vi "SMR_LabVIEW_V7.1.vi"() -> ()   [LabVIEW 2025]
uses:
  <vilib>/DAQmx/write.llb/DAQmx Write (Analog DBL 1Chan 1Samp).vi
  <vilib>/DAQmx/read.llb/DAQmx Read (Analog 1D DBL NChan 1Samp).vi
  <vilib>/DAQmx/create/channels.llb/DAQmx Create Channel (AI-Temperature-Thermocouple).vi
  <vilib>/DAQmx/create/channels.llb/DAQmx Create Channel (AI-Voltage-Basic).vi
  <vilib>/DAQmx/create/channels.llb/DAQmx Create Channel (AO-Voltage-Basic).vi
  <vilib>/DAQmx/miscellaneous.llb/DAQmx Fill In Error Info.vi
  <vilib>/addons/control/pid/pid.llb/PID (DBL).vi
  <vilib>/addons/control/pid/NI_PID_pid.lvlib
panel:
  out "Final P-Valve Voltage (V)":dbl
  out "PID Trim Voltage (V)":dbl
  in  "PID Temp Setpoint (deg C)":dbl
  in  "Auto PID Enable":bool
  in  "Manual P-Valve Voltage (V)":dbl min=0.0 max=10.0
  out "Rate Window Ready":bool
  out "Steady State":bool
  in  "Steady State Threshold (deg C/min)":dbl=0.5
  out "Temp Change Rate (deg C/min)":dbl
  in  "Voltage Limit (V)":dbl=10.0
  in  "Temperature Limit (C)":dbl=50.0
  in  "Pressure Limit (psi)":dbl=15.0
  out "Max Voltage":bool
  out "Max Temperature":bool
  out "Max Pressure":bool
  out "Current Run Folder":path
  in  "Log Root Folder":path=path "C:/Users/LocalUser/Documents/GitHub/thermal-loop/resources/v0.1.1/data/001"
  out "Heat Exchanger Pressure History":dbl(graph)
  out "Main Loop Pressure History":T1(graph)
  out "Heat Exchanger Temperature History":cluster{"Waveform":dbl, "Waveform":dbl}(graph)
  out "Main Loop Temeperature History":T2(graph)
  out "Overall Avg Pressure (psi)":dbl
  out "Heat Exchanger Pressure P6 (psi)":dbl
  out "Main Loop Avg Pressure (psi)":dbl
  out "Heat Exchanger Avg Temp (deg C)":dbl
  out "Main Loop Avg Temp (deg C)":dbl
  out "Raw NI9201 \nVoltage Display":T3
  out "Temperature Display":T4
  out "Pressure Display":T5
  in  "Flow Offset Correction (GPM)":dbl=-0.3
  out "Flow History":dbl(graph)
  out "Overall Pressure History":T6(graph)
  out "Overall Temperature History":T7(graph)
  out "Max Loop Pressure (psi)":dbl
  out "Overall Avg Temp (deg C)":dbl
  out "Max Loop Temp (deg C)":dbl
  out "Heat Exchanger Flow (GPM)":dbl
  in  "Loop Period (ms)":dbl=1000.0
  in  "Stop":bool
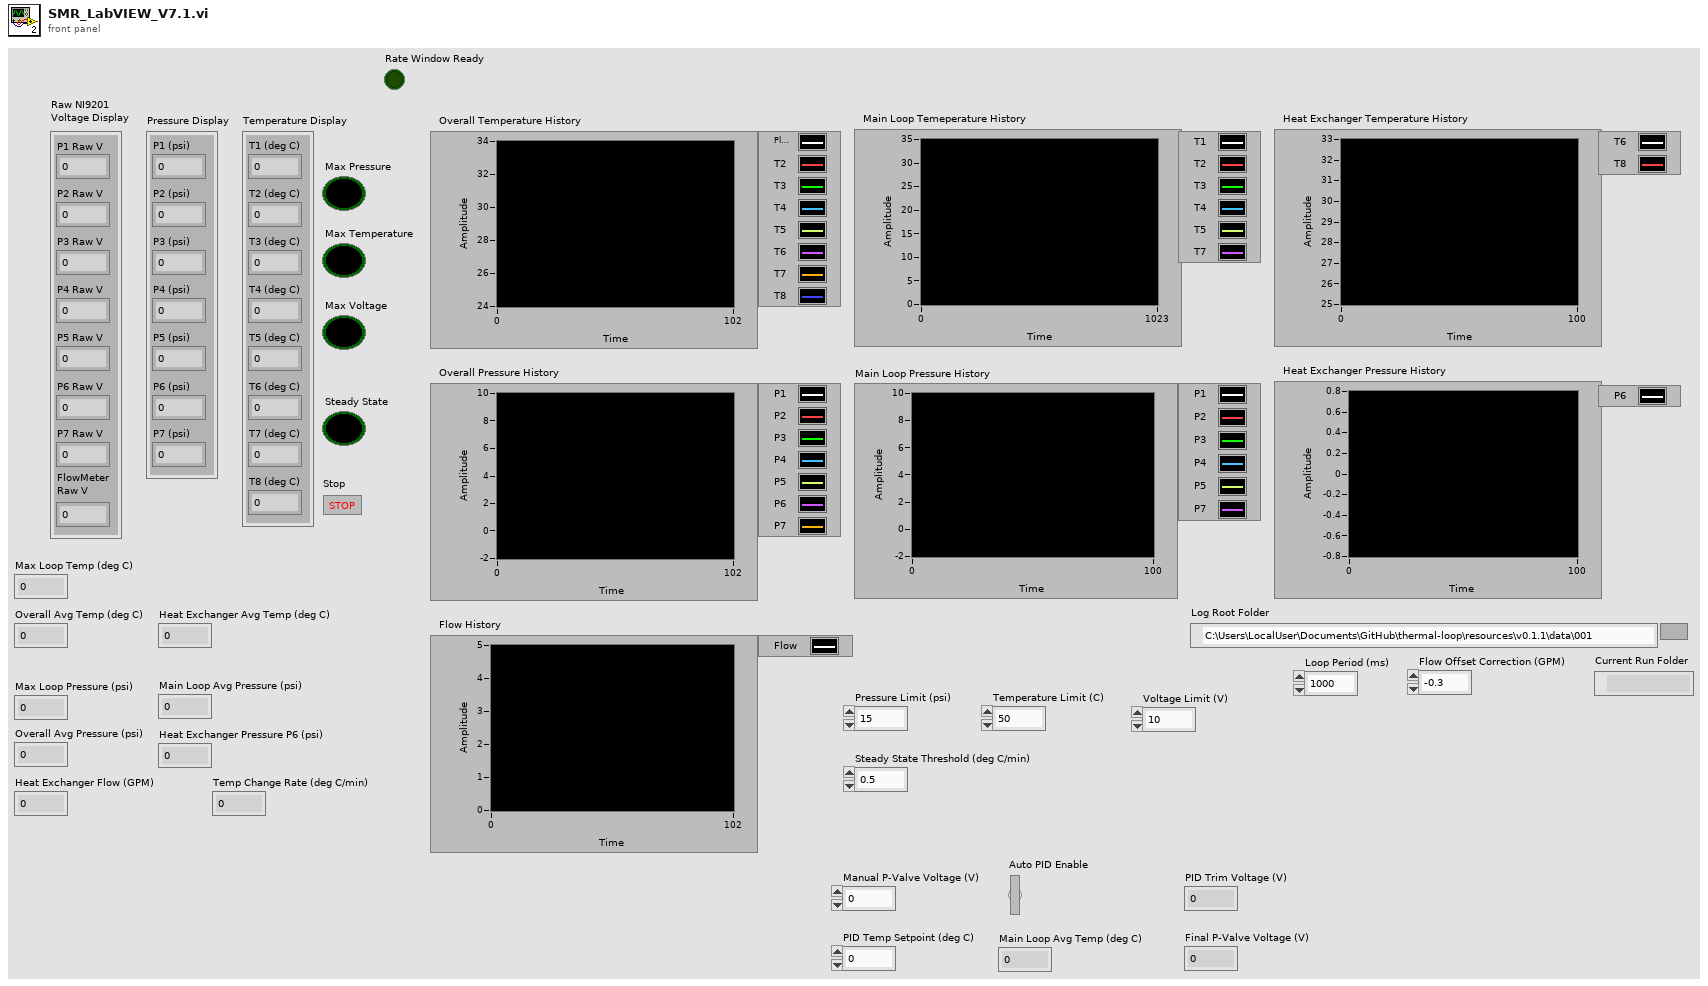
[diagram p1: front panel]
types:
  T1 = cluster{"P1":dbl, "P2":dbl, "P3":dbl, "P4":dbl, "P5":dbl, "P7":dbl}
  T2 = cluster{"Waveform":dbl, "Waveform":dbl, "Waveform":dbl, "Waveform":dbl, "Waveform":dbl, "Waveform":dbl}
  T3 = cluster{"P1 Raw V":dbl, "P2 Raw V":dbl, "P3 Raw V":dbl, "P4 Raw V":dbl, "P5 Raw V":dbl, "P6 Raw V":dbl, "P7 Raw V":dbl, "FlowMeter\nRaw V":dbl}
  T4 = cluster{"T1 (deg C)":dbl, "T2 (deg C)":dbl, "T3 (deg C)":dbl, "T4 (deg C)":dbl, "T5 (deg C)":dbl, "T6 (deg C)":dbl, "T7 (deg C)":dbl, "T8 (deg C)":dbl}
  T5 = cluster{"P1 (psi)":dbl, "P2 (psi)":dbl, "P3 (psi)":dbl, "P4 (psi)":dbl, "P5 (psi)":dbl, "P6 (psi)":dbl, "P7 (psi)":dbl}
  T6 = cluster{"P1":dbl, "P2":dbl, "P3":dbl, "P4":dbl, "P5":dbl, "P6":dbl, "P7":dbl}
  T7 = cluster{"Waveform":dbl, "Waveform":dbl, "Waveform":dbl, "Waveform":dbl, "Waveform":dbl, "Waveform":dbl, "Waveform":dbl, "Waveform":dbl}
  T8 = enum16{"open", "replace", "create", "open or create", "replace or create", "replace or create with confirmation"}
  T9 = cluster{"proportional gain (Kc)":dbl, "integral time (Ti, min)":dbl, "derivative time (Td, min)":dbl}
  T10 = cluster{"P1":dbl, "P2":dbl, "P3":dbl, "P4":dbl, "P5":dbl, "P6":dbl, "P7":dbl, "Flow":dbl}
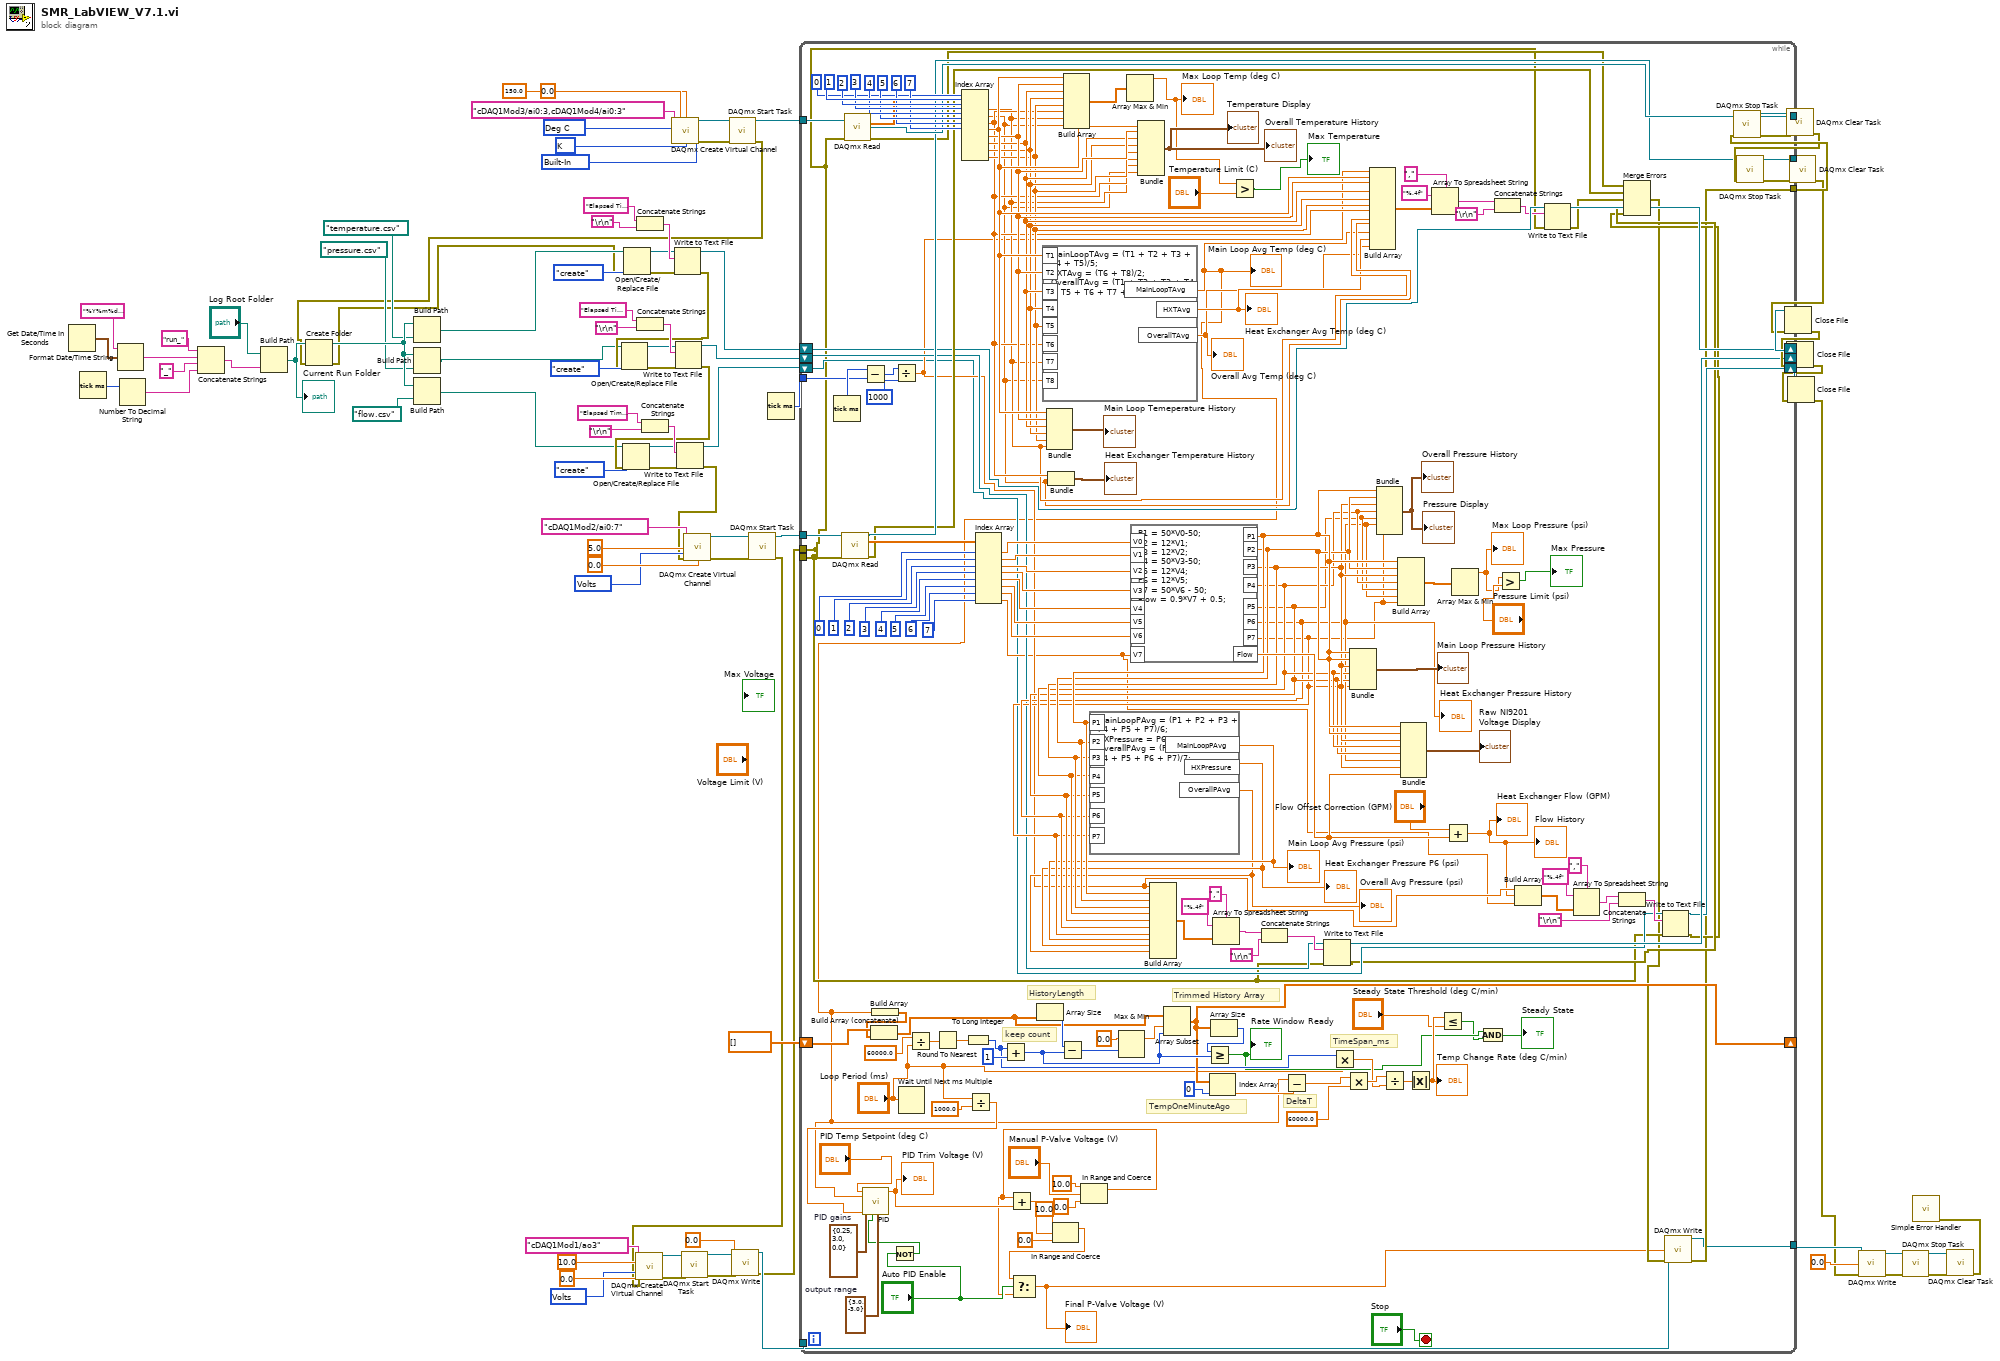
[diagram p0: block diagram]
diagram:
  w17 = 10348 items=["Volts"=10348, "From Custom Scale"=10065] ("units")
  w83 = 10200 items=["Built-In"=10200, "Constant Value"=10116, "Channel"=10113] ("cjc source")
  w84 = 10073 items=["J"=10072, "K"=10073, "N"=10077, "R"=10082, "S"=10085, "T"=10086, "B"=10047, "E"=10055] ("thermocouple type")
  w85 = 10143 items=["Deg C"=10143, "Deg F"=10144, "Kelvins"=10325, "Deg R"=10145, "From Custom Scale"=10065] ("units")
  w92 = 10348 items=["Volts"=10348, "From Custom Scale"=10065] ("units")
  n1 = Get Date/Time In Seconds() -> (seconds since 1Jan1904=w40:timestamp)
  n2 = Tick Count (ms)() -> (millisecond timer value=w38:u32)
  n3 = Format Date/Time String(time format string (%c)="%Y%m%d_%H%M%S", seconds (now)=w40) -> (date/time string=w35:string)  [unwired: 1 in]
  n4 = Number To Decimal String(number=w38) -> (decimal integer string=w36:string)  [unwired: 1 in]
  n5 = Concatenate Strings("run_" ("string"), w35, "_" ("string"), w36) -> (w32:string)
  n6 = Build Path(base path="Log Root Folder", name or relative path=w32) -> (appended path=w31:path)
  "Current Run Folder" <- w31
  n7 = Concatenate Strings("Elapsed Time (s),T1 (deg C),T2 (deg C),T3 (deg C),T4 (deg C),T5 (deg C),T6 (deg C),T7 (deg C),T8 (deg C),Main Loop Avg Temp (deg C),HX Avg Temp (deg C),Overall Avg Temp (deg C)", "\r\n") -> (w66:string)
  n8 = Concatenate Strings("Elapsed Time (s),P1 (psi),P2 (psi),P3 (psi),P4 (psi),P5 (psi),P6 (psi),P7 (psi),Main Loop Avg Pressure (psi),HX Pressure (psi),Overall Avg Pressure (psi)", "\r\n") -> (w64:string)
  n9 = Concatenate Strings("Elapsed Time (s),Heat Exchanger Flow (GPM),Flow Raw Voltage (V)", "\r\n") -> (w60:string)
  n10 = call-poly <vilib>:"DAQmx Create Virtual Channel.vi"("maximum value"=150.0, "minimum value"=0.0, "physical channels"=tag "cDAQ1Mod3/ai0:3,cDAQ1Mod4/ai0:3", "cjc source"=w83, "units"=w85, "thermocouple type"=w84) -> ("task out"=w82:refnum<k21>, "error out"=w81:errorcluster)  [unwired: 8 in]
  n11 = call <vilib>:"DAQmx Start Task.vi"("task/channels in"=w82, "error in"=w81) -> ("task out"=w80:refnum<k21>, "error out"=w23:errorcluster)  [unwired: 12 in]
  n12 = Create Folder(path (use dialog)=w31, error in=w23) -> (created path=w30:path, error out=w22:errorcluster)  [unwired: 1 in, 1 out]
  n13 = Build Path(base path=w30, name or relative path=path "temperature.csv") -> (appended path=w29:path)
  n14 = Build Path(base path=w30, name or relative path=path "pressure.csv") -> (appended path=w28:path)
  n15 = Build Path(base path=w30, name or relative path=path "flow.csv") -> (appended path=w27:path)
  n16 = Open/Create/Replace File(file path (use dialog)=w29, error in=w22, operation (0:open)=T8."create") -> (refnum out=w65:refnum<file>, error out=w49:errorcluster)  [unwired: 3 in, 1 out]
  n17 = Write to Text File(file (use dialog)=w65, text=w66, error in=w49) -> (refnum out=w56:refnum<file>, error out=w48:errorcluster)  [unwired: 1 in, 1 out]
  n18 = Open/Create/Replace File(file path (use dialog)=w28, error in=w48, operation (0:open)=T8."create") -> (refnum out=w63:refnum<file>, error out=w47:errorcluster)  [unwired: 3 in, 1 out]
  n19 = Write to Text File(file (use dialog)=w63, text=w64, error in=w47) -> (refnum out=w55:refnum<file>, error out=w46:errorcluster)  [unwired: 1 in, 1 out]
  n20 = Open/Create/Replace File(file path (use dialog)=w27, error in=w46, operation (0:open)=T8."create") -> (refnum out=w59:refnum<file>, error out=w45:errorcluster)  [unwired: 3 in, 1 out]
  n21 = Write to Text File(file (use dialog)=w59, text=w60, error in=w45) -> (refnum out=w54:refnum<file>, error out=w44:errorcluster)  [unwired: 1 in, 1 out]
  n22 = call-poly <vilib>:"DAQmx Create Virtual Channel.vi"("maximum value"=5.0, "minimum value"=0.0, "physical channels"=tag "cDAQ1Mod2/ai0:7", "units"=w92, "error in"=w44) -> ("task out"=w91:refnum<k21>, "error out"=w90:errorcluster)  [unwired: 9 in]
  n23 = call <vilib>:"DAQmx Start Task.vi"("task/channels in"=w91, "error in"=w90) -> ("task out"=w89:refnum<k21>, "error out"=w10:errorcluster)  [unwired: 12 in]
  n24 = call-poly <vilib>:"DAQmx Create Virtual Channel.vi"("maximum value"=10.0, "minimum value"=0.0, "physical channels"=tag "cDAQ1Mod1/ao3", "units"=w17, "error in"=w10) -> ("task out"=w16:refnum<k21>, "error out"=w15:errorcluster)  [unwired: 9 in]
  n25 = call <vilib>:"DAQmx Start Task.vi"("task/channels in"=w16, "error in"=w15) -> ("task out"=w14:refnum<k21>, "error out"=w13:errorcluster)  [unwired: 12 in]
  n26 = call-poly <vilib>:"DAQmx Write.vi"("task/channels in"=w14, "data"=0.0, "error in"=w13) -> ("task out"=w11:refnum<k21>, "error out"=w9:errorcluster)  [unwired: 10 in, 1 out]
  n27 = Tick Count (ms)() -> (millisecond timer value=w53:u32)
  n28 = while {
    tunnel: w89 -> [w246]
    tunnel: w80 -> [w220]
    tunnel: [w210] -> w79
    tunnel: [w116] -> _
    tunnel: [w209] -> w78
    tunnel: [w114] -> w77
    shift-right: [w186] -> w52
    shift-left: w56 -> [w187]
    shift-right: [w167] -> w51
    shift-left: w55 -> [w168]
    shift-right: [w156] -> w50
    shift-left: w54 -> [w157]
    tunnel: w53 -> [w205]
    shift-right: [w133] -> _
    shift-left: dbl[] [] -> [w146]
    tunnel: w11 -> [w106]
    tunnel: w9 -> [w116]
    tunnel: [w113] -> w7
    stop <- "Stop" stop-if-true
    w111 = cluster{"output high":dbl, "output low":dbl} {"output high"=3.0, "output low"=-3.0}  # output range
    w112 = T9 {"proportional gain (Kc)"=0.25, "integral time (Ti, min)"=3.0, "derivative time (Td, min)"=0.0}  # PID gains
    # "TimeSpan_ms"
    # "DeltaT"
    # "TempOneMinuteAgo"
    # "Trimmed History Array"
    # "HistoryLength"
    # "keep count"
    n29 = Tick Count (ms)() -> (millisecond timer value=w206:u32)
    n30 = call-poly <vilib>:"DAQmx Read.vi"("task/channels in"=w246, "error in"=w116) -> ("task out"=w209:refnum<k21>, "data"=w237:dbl[], "error out"=w207:errorcluster)  [unwired: 11 in]
    n31 = call-poly <vilib>:"DAQmx Read.vi"("task/channels in"=w220, "error in"=w116) -> ("task out"=w210:refnum<k21>, "data"=w211:dbl[], "error out"=w208:errorcluster)  [unwired: 11 in]
    n32 = Subtract(x=w206, y=w205) -> (x-y=w204:u32)
    n33 = Not(x="Auto PID Enable") -> (.not. x?=w107:bool)
    n34 = Divide(x=w204, y=u32 1000) -> (x/y=w166:dbl)
    n35 = Wait Until Next ms Multiple(millisecond multiple="Loop Period (ms)") -> ()  [unwired: 1 out]
    n36 = Divide(x=60000.0, y="Loop Period (ms)") -> (x/y=w143:dbl)
    n37 = Round To Nearest(number=w143) -> (nearest integer value=w142:dbl)
    n38 = Index Array(array=w211, index #1=0 ("index"), index #2=1 ("index"), index #3=2 ("index"), index #4=3 ("index"), index #5=4 ("index"), index #6=5 ("index"), index #7=6 ("index"), index #8=7 ("index")) -> (element #1=w196:dbl, element #2=w195:dbl, element #3=w197:dbl, element #4=w202:dbl, element #5=w201:dbl, element #6=w200:dbl, element #7=w199:dbl, element #8=w198:dbl)
    n39 = To Long Integer(number=w142) -> (32bit integer=w130:i32)
    n40 = Divide(x="Loop Period (ms)", y=1000.0) -> (x/y=w108:dbl)
    n41 = Index Array(array=w237, index #1=0 ("index"), index #2=1 ("index"), index #3=2 ("index"), index #4=3 ("index"), index #5=4 ("index"), index #6=5 ("index"), index #7=6 ("index"), index #8=7 ("index")) -> (element #1=w236:dbl, element #2=w235:dbl, element #3=w234:dbl, element #4=w233:dbl, element #5=w232:dbl, element #6=w231:dbl, element #7=w230:dbl, element #8=w164:dbl)
    n42 = Add(x=w130, y=1) -> (x+y=w135:i32)
    n43 = formula code="MainLoopTAvg = (T1 + T2 + T3 + T4 + T5)/5;\nHXTAvg = (T6 + T8)/2;\nOverallTAvg = (T1 + T2 + T3 + T4 + T5 + T6 + T7 + T8)/8;"("T1"=w202, "T2"=w201, "T3"=w200, "T4"=w199, "T5"=w198, "T6"=w197, "T7"=w196, "T8"=w195) -> ("MainLoopTAvg"=w97:dbl, "HXTAvg"=w194:dbl, "OverallTAvg"=w193:dbl)
    "Overall Avg Temp (deg C)" <- w193
    "Main Loop Avg Temp (deg C)" <- w97
    "Heat Exchanger Avg Temp (deg C)" <- w194
    n44 = call-poly <vilib>:"PID.vi"("reinitialize? (F)"=w107, "output range"=w111, "dt (s)"=w108, "PID gains"=w112, "process variable"=w97, "setpoint"="PID Temp Setpoint (deg C)") -> ("output"=w105:dbl)  [unwired: 4 in, 1 out]
    "PID Trim Voltage (V)" <- w105
    n45 = Build Array(w97) -> (w145:dbl[])
    n46 = Build Array (concatenate)(w146, w145) -> (w137:dbl[])
    n47 = Array Size(array=w137) -> (size(s)=w140:i32)
    n48 = Bundle("Waveform"=w202, "Waveform"=w201, "Waveform"=w200, "Waveform"=w199, "Waveform"=w198, "Waveform"=w196) -> (→"Main Loop Temeperature History":T2)  [unwired: 1 in]
    n49 = Bundle("Waveform"=w197, "Waveform"=w195) -> (→"Heat Exchanger Temperature History":cluster{"Waveform":dbl, "Waveform":dbl})  [unwired: 1 in]
    n50 = Subtract(x=w140, y=w135) -> (x-y=w138:i32)
    n51 = Build Array(w202, w201, w200, w199, w198, w197, w196, w195) -> (w247:dbl[])
    n52 = In Range and Coerce(upper limit=10.0, x="Manual P-Valve Voltage (V)", lower limit=0.0) -> (coerced(x)=w100:dbl)  [unwired: 1 out]
    n53 = Add(x=w100, y=w105) -> (x+y=w104:dbl)
    n54 = In Range and Coerce(upper limit=10.0, x=w104, lower limit=0.0) -> (coerced(x)=w99:dbl)  [unwired: 1 out]
    n55 = Select(t=w99, s="Auto PID Enable", f=w100) -> (s? t:f=w98:dbl)
    "Final P-Valve Voltage (V)" <- w98
    n56 = Max & Min(x=0.0, y=w138) -> (max(x,y)=w136:dbl)  [unwired: 1 out]
    n57 = Array Max & Min(array=w247) -> (max value=w149:dbl)  [unwired: 3 out]
    "Max Loop Temp (deg C)" <- w149
    n58 = formula code="P1 = 50*V0-50;\nP2 = 12*V1;\nP3 = 12*V2;\nP4 = 50*V3-50;\nP5 = 12*V4;\nP6 = 12*V5; \nP7 = 50*V6 - 50;\nFlow = 0.9*V7 + 0.5;"("V0"=w236, "V1"=w235, "V2"=w234, "V3"=w233, "V4"=w232, "V5"=w231, "V6"=w230, "V7"=w164) -> ("P1"=w185:dbl, "P2"=w184:dbl, "P3"=w183:dbl, "P4"=w182:dbl, "P5"=w181:dbl, "P6"=w180:dbl, "P7"=w179:dbl, "Flow"=w225:dbl)
    "Heat Exchanger Pressure History" <- w180
    n59 = formula code="MainLoopPAvg = (P1 + P2 + P3 + P4 + P5 + P7)/6;\nHXPressure = P6;\nOverallPAvg = (P1 + P2 + P3 + P4 + P5 + P6 + P7)/7;"("P1"=w185, "P2"=w184, "P3"=w183, "P4"=w182, "P5"=w181, "P6"=w180, "P7"=w179) -> ("MainLoopPAvg"=w178:dbl, "HXPressure"=w177:dbl, "OverallPAvg"=w176:dbl)
    "Overall Avg Pressure (psi)" <- w176
    "Heat Exchanger Pressure P6 (psi)" <- w177
    "Main Loop Avg Pressure (psi)" <- w178
    n60 = Bundle("Waveform"=w202, "Waveform"=w201, "Waveform"=w200, "Waveform"=w199, "Waveform"=w198, "Waveform"=w197, "Waveform"=w196, "Waveform"=w195) -> (→"Overall Temperature History" →"Temperature Display":T7)  [unwired: 1 in]
    n61 = Build Array(w166, w185, w184, w183, w182, w181, w180, w179, w178, w177, w176) -> (w175:dbl[])
    n62 = Array Subset(array=w137, index=w136, length=w135) -> (w133:dbl[])
    n63 = Index Array(array=w133, index=0) -> (element=w131:dbl)
    n64 = Array Size(array=w133) -> (size(s)=w134:i32)
    n65 = Greater Or Equal?(x=w134, y=w135) -> (x >= y?=w122:bool)
    "Rate Window Ready" <- w122
    n66 = Array To Spreadsheet String(delimiter (Tab)=",", array=w175, 3:"%.4f" ("format string")) -> (spreadsheet string=w171:string)
    n67 = Greater?(x=w149, y="Temperature Limit (C)") -> (0:→"Max Temperature":bool)
    n68 = Concatenate Strings(w171, "\r\n") -> (w169:string)
    n69 = Subtract(x=w97, y=w131) -> (x-y=w129:dbl)
    n70 = Write to Text File(file (use dialog)=w168, text=w169, error in=w116) -> (refnum out=w167:refnum<file>, error out=w154:errorcluster)  [unwired: 1 in, 1 out]
    n71 = Multiply(x=w130, y="Loop Period (ms)") -> (x*y=w126:dbl)
    n72 = Multiply(x=w129, y=60000.0) -> (x*y=w127:dbl)
    n73 = Bundle("P1"=w185, "P2"=w184, "P3"=w183, "P4"=w182, "P5"=w181, "P7"=w179) -> (→"Main Loop Pressure History":T1)  [unwired: 1 in]
    n74 = Build Array(w166, w202, w201, w200, w199, w198, w197, w196, w195, w97, w194, w193) -> (w192:dbl[])
    n75 = Bundle("P1"=w185, "P2"=w184, "P3"=w183, "P4"=w182, "P5"=w181, "P6"=w180, "P7"=w179) -> (→"Overall Pressure History" →"Pressure Display":T6)  [unwired: 1 in]
    n76 = Divide(x=w127, y=w126) -> (x/y=w125:dbl)
    n77 = Build Array(w185, w184, w183, w182, w181, w180, w179) -> (w228:dbl[])
    n78 = Bundle("P1"=w185, "P2"=w184, "P3"=w183, "P4"=w182, "P5"=w181, "P6"=w180, "P7"=w179, "Flow"=w225) -> (→"Raw NI9201 \nVoltage Display":T10)  [unwired: 1 in]
    n79 = Absolute Value(x=w125) -> (abs(x)=w124:dbl)
    "Temp Change Rate (deg C/min)" <- w124
    n80 = Array To Spreadsheet String(delimiter (Tab)=",", array=w192, 3:"%.4f" ("format string")) -> (spreadsheet string=w189:string)
    n81 = Less Or Equal?(x=w124, y="Steady State Threshold (deg C/min)") -> (x <= y?=w121:bool)
    n82 = Add(x="Flow Offset Correction (GPM)", y=w225) -> (x+y=w165:dbl)
    "Heat Exchanger Flow (GPM)" <- w165
    "Flow History" <- w165
    n83 = Array Max & Min(array=w228) -> (max value=w151:dbl)  [unwired: 3 out]
    "Max Loop Pressure (psi)" <- w151
    n84 = And(x=w122, y=w121) -> (x .and. y?=→"Steady State":bool)
    n85 = Concatenate Strings(w189, "\r\n") -> (w172:string)
    n86 = Greater?(x=w151, y="Pressure Limit (psi)") -> (0:→"Max Pressure":bool)
    n87 = Build Array(w166, w165, w164) -> (w163:dbl[])
    n88 = Write to Text File(file (use dialog)=w187, text=w172, error in=w116) -> (refnum out=w186:refnum<file>, error out=w155:errorcluster)  [unwired: 1 in, 1 out]
    n89 = Array To Spreadsheet String(delimiter (Tab)=",", array=w163, 3:"%.4f" ("format string")) -> (spreadsheet string=w159:string)
    n90 = Concatenate Strings(w159, "\r\n") -> (w158:string)
    n91 = Write to Text File(file (use dialog)=w157, text=w158, error in=w116) -> (refnum out=w156:refnum<file>, error out=w153:errorcluster)  [unwired: 1 in, 1 out]
    n92 = Merge Errors(w208, w207, w155, w154, w153) -> (w115:errorcluster)
    n93 = call-poly <vilib>:"DAQmx Write.vi"("task/channels in"=w106, "data"=w98, "error in"=w115) -> ("task out"=w113:refnum<k21>, "error out"=w114:errorcluster)  [unwired: 10 in, 1 out]
  }
  n94 = call <vilib>:"DAQmx Stop Task.vi"("task/channels in"=w79, "error in"=w77) -> ("task out"=w76:refnum<k21>, "error out"=w74:errorcluster)  [unwired: 12 in]
  n95 = call <vilib>:"DAQmx Clear Task.vi"("task in"=w76, "error in"=w74) -> ("error out"=w73:errorcluster)  [unwired: 13 in]
  n96 = call <vilib>:"DAQmx Stop Task.vi"("task/channels in"=w78, "error in"=w73) -> ("task out"=w75:refnum<k21>, "error out"=w72:errorcluster)  [unwired: 12 in]
  n97 = call <vilib>:"DAQmx Clear Task.vi"("task in"=w75, "error in"=w72) -> ("error out"=w43:errorcluster)  [unwired: 13 in]
  n98 = Close File(refnum=w52, error in=w43) -> (error out=w42:errorcluster)  [unwired: 1 out]
  n99 = Close File(refnum=w51, error in=w42) -> (error out=w41:errorcluster)  [unwired: 1 out]
  n100 = Close File(refnum=w50, error in=w41) -> (error out=w6:errorcluster)  [unwired: 1 out]
  n101 = call-poly <vilib>:"DAQmx Write.vi"("task/channels in"=w7, "data"=0.0, "error in"=w6) -> ("task out"=w5:refnum<k21>, "error out"=w3:errorcluster)  [unwired: 10 in, 1 out]
  n102 = call <vilib>:"DAQmx Stop Task.vi"("task/channels in"=w5, "error in"=w3) -> ("task out"=w4:refnum<k21>, "error out"=w2:errorcluster)  [unwired: 12 in]
  n103 = call <vilib>:"DAQmx Clear Task.vi"("task in"=w4, "error in"=w2) -> ("error out"=w1:errorcluster)  [unwired: 13 in]
  n104 = call <vilib>:"Simple Error Handler.vi"("error in (no error)"=w1) -> ()  [unwired: 4 in, 5 out]
